vi "Q.Enqueue Data.vi"(4 "Data2":variant, 5 "Top of Q":bool, 6 "Data1":variant, 7 "Q Name":string, 8 "Error In":errorcluster, 9 "Seq Task Name":string, 11 "Q In":refnum<queue>) -> (0 "error out":errorcluster, 3 "Q Out":refnum<queue>)   [LabVIEW 2024, in "EQMF.lvlib" / "Queue Utils.lvlib"]
doc: "This VI enqueues a Task:\n Queue element 'Cmd' = \"Task\"\n Queue element 'Sub' is assigned to the value of the 'Task Name' input.\n\nThis VI obtains the queue by name or by queue reference.\nIf the 'Q Name' input is empty then it obtains the queue by the 'Q In\" reference.\nIf the 'Q Name' input is NOT empty then it obtains the queue by the this name.\n If a queue is ontained by name and the queue does not already exits, an error is generated.\n\nThe 'Top of Q' input is FALSE by default.\nThis input will cause this item to be enqueued on the top of the queue when it is TRUE."
uses:
  Queue Utils.lvlib
  Q.Element.ctl
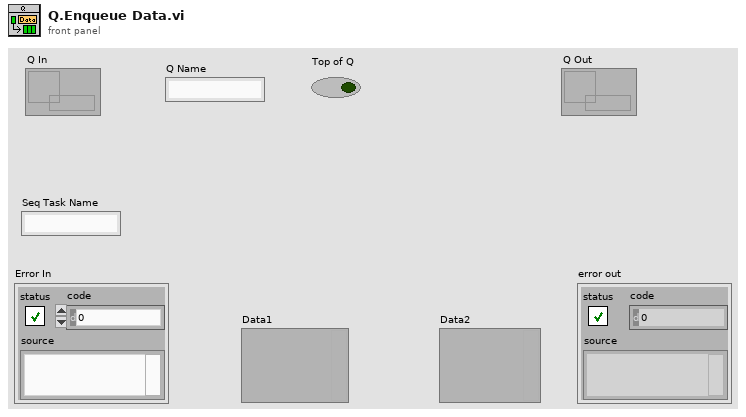
[diagram p1: front panel]
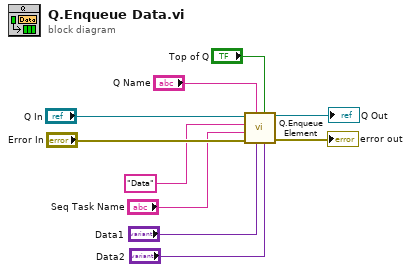
[diagram p0: block diagram]
diagram:
  n1 = call "Q.Enqueue Element.vi"("Data2"="Data2", "Top of Q"="Top of Q", "Data1"="Data1", "Q Name"="Q Name", "error in"="Error In", "Sub"="Seq Task Name", "Cmd"="Data", "Q In"="Q In") -> ("error out"=→"error out":errorcluster, "Q Out"=→"Q Out":refnum<queue>)  [unwired: 2 in]
